vi "swerve_math.vi"(0 "FWD":dbl(slide) scale=-1.0..1.0, 2 "STR":dbl(slide) scale=-1.0..1.0, 4 "RCW":dbl(slide) scale=-1.0..1.0) -> (20 "Power FL":dbl, 21 "Steering FL":dbl, 22 "Power FR":dbl, 23 "Steering FR":dbl, 24 "Power BL":dbl, 25 "Steering BL":dbl, 26 "Power BR":dbl, 27 "Steering BR":dbl)   [LabVIEW 2020]
panel:
  out "Back Right":cluster{"X":dbl, "Y":dbl}[](graph)
  out "Back Left":cluster{"X":dbl, "Y":dbl}[](graph)
  out "Front Right":cluster{"X":dbl, "Y":dbl}[](graph)
  out "Front Left":cluster{"X":dbl, "Y":dbl}[](graph)
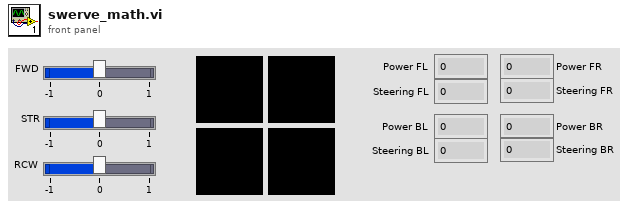
[diagram p1: front panel]
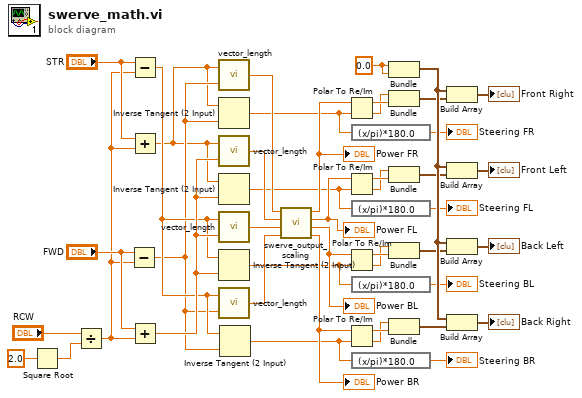
[diagram p0: block diagram]
diagram:
  w38 = 0.0 ("x")
  n1 = Square Root(x=2.0) -> (sqrt(x)=w44:dbl)
  n2 = Divide(x="RCW", y=w44) -> (x/y=w39:dbl)
  n3 = Subtract(x="FWD", y=w39) -> (x-y=w10:dbl)
  n4 = Subtract(x="STR", y=w39) -> (x-y=w11:dbl)
  n5 = Add(x="STR", y=w39) -> (x+y=w9:dbl)
  n6 = Add(x="FWD", y=w39) -> (x+y=w12:dbl)
  n7 = call "vector_length.vi"("v_y"=w10, "v_x"=w9) -> ("||v||"=w28:dbl)
  n8 = Inverse Tangent (2 Input)(1:w10, 2:w9) -> (0:w17:dbl)
  n9 = call "vector_length.vi"("v_y"=w12, "v_x"=w9) -> ("||v||"=w27:dbl)
  n10 = Inverse Tangent (2 Input)(1:w12, 2:w9) -> (0:w18:dbl)
  n11 = call "vector_length.vi"("v_y"=w12, "v_x"=w11) -> ("||v||"=w26:dbl)
  n12 = Inverse Tangent (2 Input)(1:w12, 2:w11) -> (0:w19:dbl)
  n13 = call "vector_length.vi"("v_y"=w10, "v_x"=w11) -> ("||v||"=w25:dbl)
  n14 = Inverse Tangent (2 Input)(1:w10, 2:w11) -> (0:w20:dbl)
  n15 = call "swerve_output_scaling.vi"("d"=w25, "c"=w26, "b"=w27, "a"=w28) -> ("d scaled"=w21:dbl, "c scaled"=w22:dbl, "b scaled"=w23:dbl, "a scaled"=w24:dbl)  [unwired: 4 in]
  "Power FR" <- w24
  "Power FL" <- w23
  "Power BL" <- w22
  "Power BR" <- w21
  n16 = Polar To Re/Im(2:w17, 3:w24) -> (0:w7:dbl, 1:w8:dbl)
  n17 = Polar To Re/Im(2:w18, 3:w23) -> (0:w5:dbl, 1:w6:dbl)
  n18 = Polar To Re/Im(2:w19, 3:w22) -> (0:w3:dbl, 1:w4:dbl)
  n19 = Polar To Re/Im(2:w20, 3:w21) -> (0:w1:dbl, 1:w2:dbl)
  n20 = expression code="(x/pi)*180.0" ("radians to degrees")(w17) -> (→"Steering FR":dbl)
  n21 = expression code="(x/pi)*180.0" ("radians to degrees")(w18) -> (→"Steering FL":dbl)
  n22 = expression code="(x/pi)*180.0" ("radians to degrees")(w19) -> (→"Steering BL":dbl)
  n23 = expression code="(x/pi)*180.0" ("radians to degrees")(w20) -> (→"Steering BR":dbl)
  n24 = Bundle("x"=w38, "x"=w38) -> (w37:cluster{"x":dbl, "x":dbl})  [unwired: 1 in]
  n25 = Bundle(w7, w8) -> (w31:cluster{dbl, dbl})  [unwired: 1 in]
  n26 = Bundle(w5, w6) -> (w32:cluster{dbl, dbl})  [unwired: 1 in]
  n27 = Bundle(w3, w4) -> (w30:cluster{dbl, dbl})  [unwired: 1 in]
  n28 = Bundle(w1, w2) -> (w29:cluster{dbl, dbl})  [unwired: 1 in]
  n29 = Build Array(w37, w31) -> (→"Front Right":cluster{"x":dbl, "x":dbl}[])
  n30 = Build Array(w37, w32) -> (→"Front Left":cluster{"x":dbl, "x":dbl}[])
  n31 = Build Array(w37, w30) -> (→"Back Left":cluster{"x":dbl, "x":dbl}[])
  n32 = Build Array(w37, w29) -> (→"Back Right":cluster{"x":dbl, "x":dbl}[])
